vi "Bit Rate.vi"() -> ()   [LabVIEW 2016]
uses:
  Set Save Object Dictionary.vi
  Motor controllers.vi
  <vilib>/CANopenLib/CANOPEN.llb/CANopen SDO Create.vi
  <vilib>/CANopenLib/CANOPEN.llb/CANopen SDO Write.vi
  <vilib>/CANopenLib/CANOPEN.llb/CANopen SDO Write [STR].vi
  <vilib>/CANopenLib/CANOPEN.llb/CANopen SDO Close.vi
  Get Node ID.vi
  <vilib>/CANopenLib/CANOPEN.llb/CANopen Interface Close.vi
panel:
  in  "Motor":u8(ring) items=["Right", "Left"]
  in  "New Node ID":u8=1 min=1 max=127 step=1
  out "error out":errorcluster
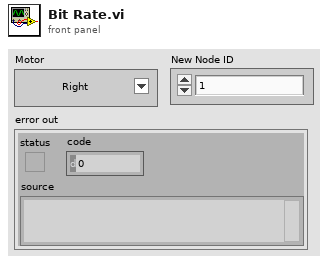
[diagram p1: front panel]
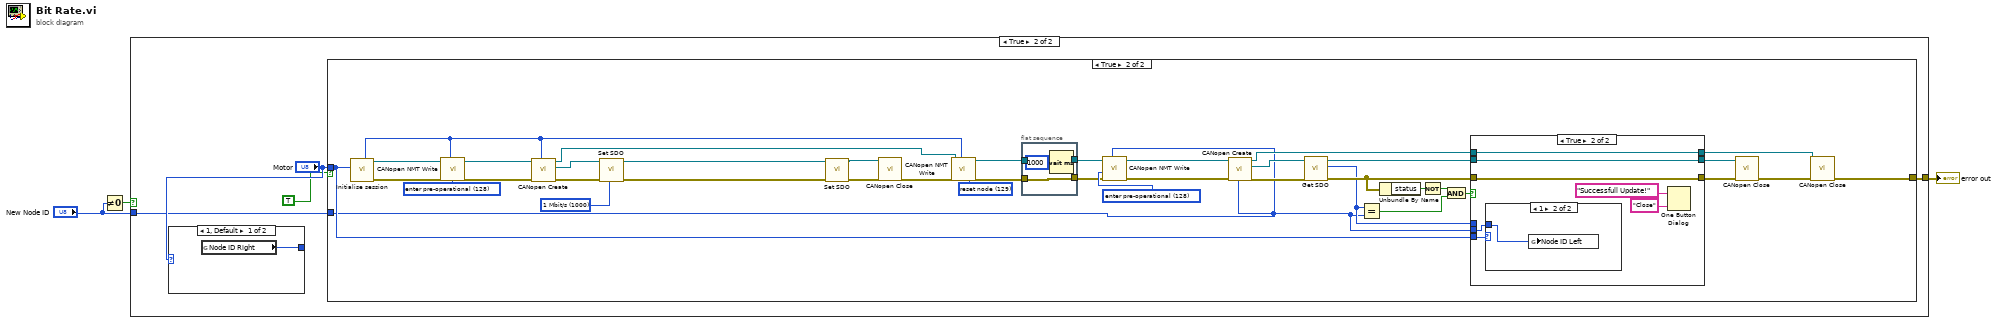
[diagram p0: block diagram]
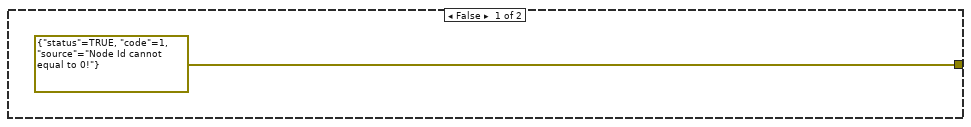
[diagram p2: hidden frame]
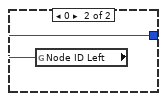
[diagram p3: hidden frame]
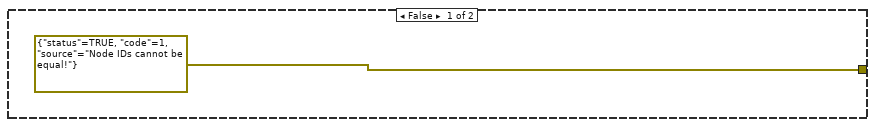
[diagram p4: hidden frame]
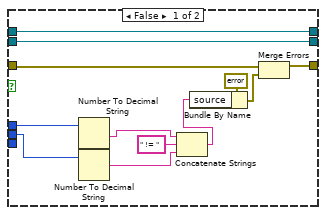
[diagram p5: hidden frame]
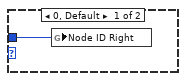
[diagram p6: hidden frame]
diagram:
  n1 = Not Equal To 0?(x="New Node ID") -> (x != 0?=w2:bool)
  n2 = case shown="True" w2 {
    tunnel: [errorcluster {"status"=TRUE, "code"=1, "source"="Node Id cannot equal to 0!"} ("error constant") w8] -> w3
    tunnel: "New Node ID" -> [_ w6]
    frame False {
    }
    frame True {
      n3 = case shown="1, Default" "Motor" {
        tunnel: [w9 w10] -> _
        frame 1, Default {
          n4 = global read "Motor controllers.vi" "Node ID Right"() -> (w9:u8)
        }
        frame 0 {
          n5 = global read "Motor controllers.vi" "Node ID Left"() -> (w10:u8)
        }
      }
      n6 = case shown="True" TRUE {
        tunnel: "Motor" -> [_ w48]
        tunnel: w6 -> [_ w19]
        tunnel: [errorcluster {"status"=TRUE, "code"=1, "source"="Node IDs cannot be equal!"} ("error constant") w34] -> w8
        frame False {
        }
        frame True {
          w14 = u16 1000 items=["1 Mbit/s"=1000, "800 kbit/s"=800, "500 kbit/s"=500, "250 kbit/s"=250, "125 kbit/s"=125, "50 kbit/s"=50, "20 kbit/s"=20] ("New Baud Rate")
          w20 = u16 128 items=["start remote node"=1, "stop remote node"=2, "enter pre-operational"=128, "reset node"=129, "reset communication"=130] ("command")
          w21 = u16 129 items=["start remote node"=1, "stop remote node"=2, "enter pre-operational"=128, "reset node"=129, "reset communication"=130] ("command")
          w49 = u16 128 items=["start remote node"=1, "stop remote node"=2, "enter pre-operational"=128, "reset node"=129, "reset communication"=130] ("command")
          n7 = call "Initialise session.vi"("Motor"=w48) -> ("error out"=w43:errorcluster, "interface object out"=w42:refnum<k20>, "Used Node ID"=w25:u8)  [unwired: 8 in]
          n8 = call <vilib>:"CANopen NMT Write.vi"("node-ID (0)"=w25, "error in (no error)"=w43, "command"=w49, "interface object in"=w42) -> ("error out"=w45:errorcluster, "interface object out"=w44:refnum<k20>)  [unwired: 6 in]
          n9 = call-poly <vilib>:"CANopen Create.vi"("node-ID"=w25, "error in (no error)"=w45, "interface object in"=w44) -> ("error out"=w51:errorcluster, "SDO object out"=w50:refnum<k20>, "interface object out"=w22:refnum<k20>)  [unwired: 6 in]
          n10 = call-poly "Set SDO.vi"("New Baud Rate"=w14, "error in (no error)"=w51, "SDO object in"=w50) -> ("error out"=w12:errorcluster, "SDO object out"=w13:refnum<k20>)  [unwired: 6 in, 1 out]
          n11 = call-poly "Set SDO.vi"("error in (no error)"=w12, "SDO object in"=w13) -> ("error out"=w27:errorcluster, "SDO object out"=w28:refnum<k20>)  [unwired: 7 in, 1 out]
          n12 = call-poly <vilib>:"CANopen Close.vi"("error in (no error)"=w27, "SDO object in"=w28) -> ("error out"=w26:errorcluster)  [unwired: 9 in]
          n13 = call <vilib>:"CANopen NMT Write.vi"("node-ID (0)"=w25, "error in (no error)"=w26, "command"=w21, "interface object in"=w22) -> ("error out"=w15:errorcluster, "interface object out"=w17:refnum<k20>)  [unwired: 6 in]
          n14 = flat-sequence {
            tunnel: [w54] -> w18
            tunnel: w17 -> [w54]
            tunnel: [w53] -> w16
            tunnel: w15 -> [w53]
            frame #0 {
              n15 = Wait (ms)(milliseconds to wait=u32 1000) -> ()  [unwired: 1 out]
            }
          }
          n16 = call <vilib>:"CANopen NMT Write.vi"("node-ID (0)"=w19, "error in (no error)"=w16, "command"=w20, "interface object in"=w18) -> ("error out"=w23:errorcluster, "interface object out"=w24:refnum<k20>)  [unwired: 6 in]
          n17 = call-poly <vilib>:"CANopen Create.vi"("node-ID"=w19, "error in (no error)"=w23, "interface object in"=w24) -> ("error out"=w46:errorcluster, "SDO object out"=w47:refnum<k20>, "interface object out"=w31:refnum<k20>)  [unwired: 6 in]
          n18 = call-poly "Get SDO.vi"("error in (no error)"=w46, "SDO object in"=w47) -> ("error out"=w37:errorcluster, "Node ID"=w29:u8, "SDO object out"=w38:refnum<k20>)  [unwired: 6 in, 1 out]
          n19 = Equal?(x=w29, y=w19) -> (x = y?=w40:bool)
          n20 = Unbundle By Name(w37) -> ("status"=w30:bool)
          n21 = Not(x=w30) -> (.not. x?=w41:bool)
          n22 = And(x=w41, y=w40) -> (x .and. y?=w39:bool)
          n23 = case shown="True" w39 {
            tunnel: [w66 w67] -> w36
            tunnel: w48 -> [_ w73]
            tunnel: w19 -> [w59 w72]
            tunnel: w38 -> [w65 w68]
            tunnel: w37 -> [w63 w67]
            tunnel: [w65 w68] -> w33
            tunnel: [w64 w69] -> w32
            tunnel: w31 -> [w64 w69]
            tunnel: w29 -> [w60 _]
            frame False {
              n24 = Number To Decimal String(number=w60) -> (decimal integer string=w57:string)  [unwired: 1 in]
              n25 = Number To Decimal String(number=w59) -> (decimal integer string=w56:string)  [unwired: 1 in]
              n26 = Concatenate Strings(w57, " != " ("string"), w56) -> (w55:string)
              n27 = Bundle By Name(cluster=errorcluster {"status"=TRUE, "code"=1, "source"=""} ("error constant"), "source"=w55) -> (w61:errorcluster)
              n28 = Merge Errors(w63, w61) -> (w66:errorcluster)
            }
            frame True {
              n29 = case shown="1" w73 {
                tunnel: w72 -> [w74 w75]
                frame 0, Default {
                  n30 = global write "Motor controllers.vi" "Node ID Right"(w74) -> ()
                }
                frame 1 {
                  n31 = global write "Motor controllers.vi" "Node ID Left"(w75) -> ()
                }
              }
              n32 = One Button Dialog(message="Successfull Update!", button name ("OK")="Close") -> ()  [unwired: 1 out]
            }
          }
          n33 = call-poly <vilib>:"CANopen Close.vi"("error in (no error)"=w36, "SDO object in"=w33) -> ("error out"=w35:errorcluster)  [unwired: 9 in]
          n34 = call-poly <vilib>:"CANopen Close.vi"("error in (no error)"=w35, "interface object in"=w32) -> ("error out"=w34:errorcluster)  [unwired: 9 in]
        }
      }
    }
  }
  "error out" <- w3
